vi "Status-get.vi"(0 "Process in":refnum<vi>, 11 "error in (no error)":errorcluster) -> (4 "Process out":refnum<vi>, 6 "Stabilizing":bool, 8 "Measuring":bool, 10 "Lambda":bool, 15 "error out":errorcluster)   [LabVIEW 2016]
uses:
  controls/process.ctl
  <vilib>/silver_ctls/ArrayMatrixCluster/Real Matrix NI_Silver.ctl
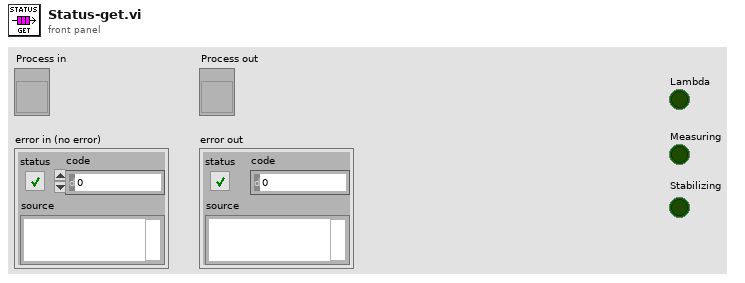
[diagram p1: front panel]
types:
  T1 = typedef "process.ctl" = cluster{"Sample":u16, "Lambda":u16, "Stabilizing":u16, "Status":u8, "Estimated Time":dbl, "Samples":T2, "Data":T2, "Lambda-Index":dbl, "Graph":bool}
  T2 = typedef "Real Matrix NI_Silver.ctl" = dbl[][]
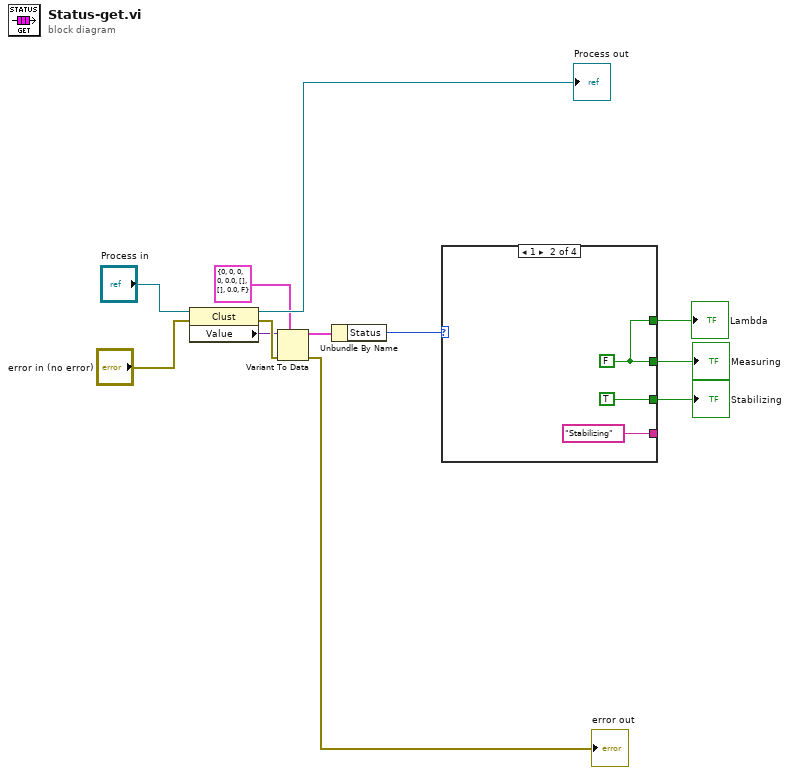
[diagram p0: block diagram]
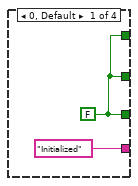
[diagram p2: hidden frame]
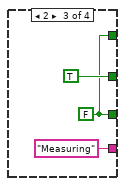
[diagram p3: hidden frame]
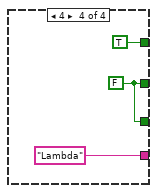
[diagram p4: hidden frame]
diagram:
  n1 = property class="Clust"(reference="Process in", error in="error in (no error)") -> (reference out=→"Process out":refnum<vi>, error out=w8:errorcluster, "Value"=w6:variant)
  n2 = Variant To Data(error in=w8, type=T1 {"Sample"=0, "Lambda"=0, "Stabilizing"=0, "Status"=0, "Estimated Time"=0.0, "Samples"=[], "Data"=[], "Lambda-Index"=0.0, "Graph"=FALSE} ("Process"), Variant=w6) -> (data=w5:T1, error out=→"error out":errorcluster)
  n3 = Unbundle By Name(w5) -> ("Status"=w4:u8)
  n4 = case shown="1" w4 {
    tunnel: ["Initialized" "Stabilizing" "Measuring" "Lambda"] -> _
    tunnel: [w13 TRUE w18 w21] -> w3
    tunnel: [w13 w15 TRUE w21] -> w2
    tunnel: [w13 w15 w18 TRUE] -> w1
    frame 0, Default {
      w13 = FALSE
    }
    frame 1 {
      w15 = FALSE
    }
    frame 2 {
      w18 = FALSE
    }
    frame 4 {
      w21 = FALSE
    }
  }
  "Stabilizing" <- w3
  "Measuring" <- w2
  "Lambda" <- w1
